vi "Memory.Pointer.Check If Equal Size.vi"(8 "error in (no error)":errorcluster, 10 "pointer b in":refnum<class "Memory.Pointer.lvclass">, 11 "pointer a in":refnum<class "Memory.Pointer.lvclass">) -> (0 "error out":errorcluster, 1 "equal size?":bool, 2 "pointer b out":refnum<class "Memory.Pointer.lvclass">, 3 "pointer a out":refnum<class "Memory.Pointer.lvclass">)   [LabVIEW 2016, in "Memory.lvlib" / "Memory.Pointer.lvclass"]
uses:
  Memory.Pointer.lvclass
  Memory.Pointer.lvclass/Memory.Pointer.ctl
  Memory.Pointer.Errors.Size Mismatch.vi
  Memory.Pointer.Errors.Create Error.vi
  Submodules/SEH/Source/VIs/Static Error Handling.Source Buffer.Write.Numeric.Scalar.Base10.vi
  Submodules/SEH/Source/VIs/Static Error Handling.Source Buffer.Write.Numeric.Scalar.Base10 (U64).vi
  Submodules/SEH/Source/VIs/Static Error Handling.Source Buffer.Write.String.vi
  Submodules/SEH/Source/VIs/Static Error Handling.Error Cluster Constant.vi
  Submodules/SEH/Source/VIs/Static Error Handling.Error Cluster Constant (256B).vi
  Submodules/SEH/Source/VIs/Static Error Handling.Parameters.Status.Set.vi
  Submodules/SEH/Source/VIs/Static Error Handling.Parameters.Code.Set.vi
  Submodules/SEH/Source/VIs/Static Error Handling.Parameters.VI Source.Set.vi
  Constants/Memory.Constants.vi
  Constants/Memory.Constants.Library Name.vi
  Memory.Pointer.Errors.Get Info.vi
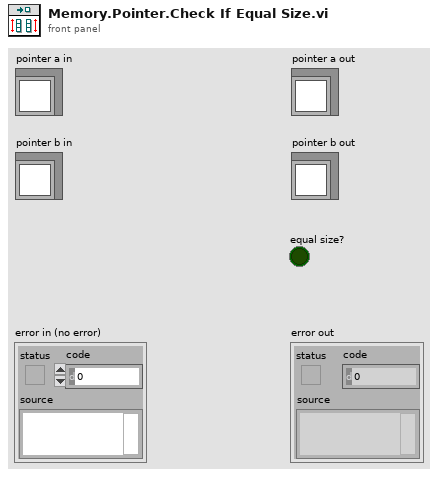
[diagram p1: front panel]
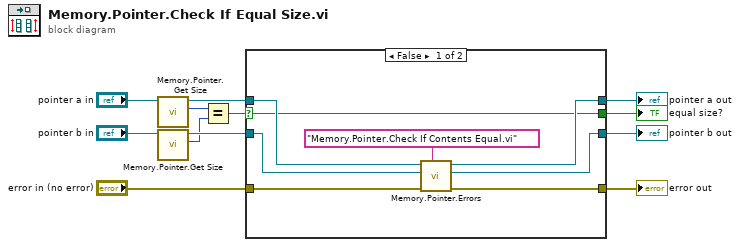
[diagram p0: block diagram]
diagram:
  n1 = call "Memory.Pointer.Get Size.vi"("Pointer in"="pointer a in") -> ("size"=w10:u64, "Pointer out"=w9:refnum<class "Memory.Pointer.lvclass">)  [unwired: 9 in]
  n2 = call "Memory.Pointer.Get Size.vi"("Pointer in"="pointer b in") -> ("size"=w6:u64, "Pointer out"=w8:refnum<class "Memory.Pointer.lvclass">)  [unwired: 9 in]
  n3 = Equal?(x=w10, y=w6) -> (x = y?=w7:bool)
  n4 = case shown="False" w7 {
    selector: w7 -> [w14 w22]
    tunnel: w9 -> [w17 w24]
    tunnel: w8 -> [w13 w23]
    tunnel: "error in (no error)" -> [w19 w21]
    tunnel: [w18 w21] -> w4
    tunnel: [w15 w24] -> w3
    tunnel: [w16 w23] -> w2
    tunnel: [w14 w22] -> w1
    frame False {
      n5 = call-poly "Memory.Pointer.Errors.vi"("source vi name"="Memory.Pointer.Check If Contents Equal.vi", "error in (no error)"=w19, "pointer b in"=w13, "pointer a in"=w17) -> ("error out"=w18:errorcluster, "pointer b out"=w16:refnum<class "Memory.Pointer.lvclass">, "pointer a out"=w15:refnum<class "Memory.Pointer.lvclass">)  [unwired: 5 in]
    }
    frame True {
    }
  }
  "error out" <- w4
  "equal size?" <- w1
  "pointer a out" <- w3
  "pointer b out" <- w2
